vi "uTTA_OpenCOM.vi"(8 "error in":errorcluster, 11 "VISA in":refnum<visa-resource-name>) -> (0 "error out":errorcluster, 2 "Identity":string, 3 "VISA out":refnum<visa-resource-name>)   [LabVIEW 2021]
uses:
  <vilib>/Instr/_visa.llb/VISA Configure Serial Port (Instr).vi
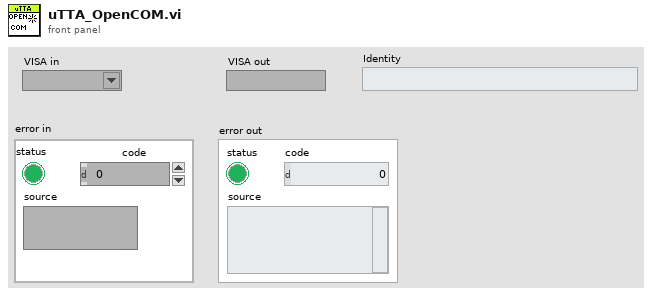
[diagram p1: front panel]
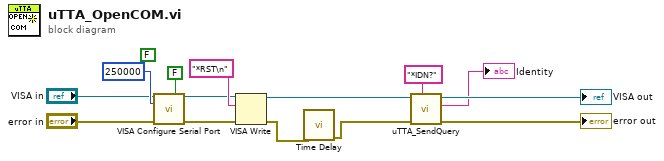
[diagram p0: block diagram]
diagram:
  (unwired) FALSE ("Enable Termination\nChar (T)")
  n1 = call-poly "VISA Configure Serial Port"("VISA resource name"="VISA in", "Enable Termination\nChar (T)"=FALSE ("Enable Termination\nChar (T)"), "baud rate (9600)"=u32 250000, "error in (no error)"="error in") -> ("VISA resource name out"=w11:refnum<visa-resource-name>, "error out"=w12:errorcluster)  [unwired: 10 in]
  n2 = VISA Write(VISA resource name=w11, write buffer="*RST\n", error in (no error)=w12) -> (VISA resource name out=w5:refnum<visa-resource-name>, error out=w14:errorcluster)  [unwired: 1 out]
  n3 = call "Time Delay"("error in (no error)"=w14) -> ("error out"=w4:errorcluster)  [unwired: 10 in]
  n4 = call "uTTA_SendQuery.vi"("Send String"="*IDN?" ("write buffer"), "error in (no error)"=w4, "VISA Refnum in"=w5) -> ("error out"=→"error out":errorcluster, "Received"=→"Identity":string, "VISA Refnum out"=→"VISA out":refnum<visa-resource-name>)  [unwired: 6 in]
